vi "DriverStationGetData.vi"   [LabVIEW 2020]
doc: "This VI recieves data from the FRC 4265 Dashboard continuously, in all robot modes. These may include safety overrides, calibration commands, and configuration parameters. However this VI should never include standard driver or manipulator commands."
uses:
  f2972b46-d919-4210-bfdf-d3cf9c7f3ddc.vi
  <vilib>/Rock Robotics/Network Tables/NT Read Boolean.vi
  driverdata.vi
  <vilib>/Rock Robotics/Network Tables/NT Read Number.vi
  sensordata.vi
  <vilib>/Rock Robotics/Network Tables/NT Read Numeric Array.vi
  refnumbers.vi
  GRNF_Joystick.vi
  <vilib>/Rock Robotics/Network Tables/NT Read String.vi
  <vilib>/Utility/xml.llb/Write to XML File(string).vi
types:
  T1 = enum16{"Center", "North", "NorthWest", "West", "SouthWest", "South", "SouthEast", "East", "NorthEast"}
  T2 = typedef "WPI_JoystickDevRef.ctl" = cluster{"Device":T3}
  T3 = typedef "WPI_JoystickDeviceEnum.ctl" = enum16{"USB 0", "USB 1", "USB 2", "USB 3", "USB 4", "USB 5"}
  T4 = typedef "WPI_DriverStationAllianceInfo.ctl" = enum16{"Red", "Blue", "Invalid"}
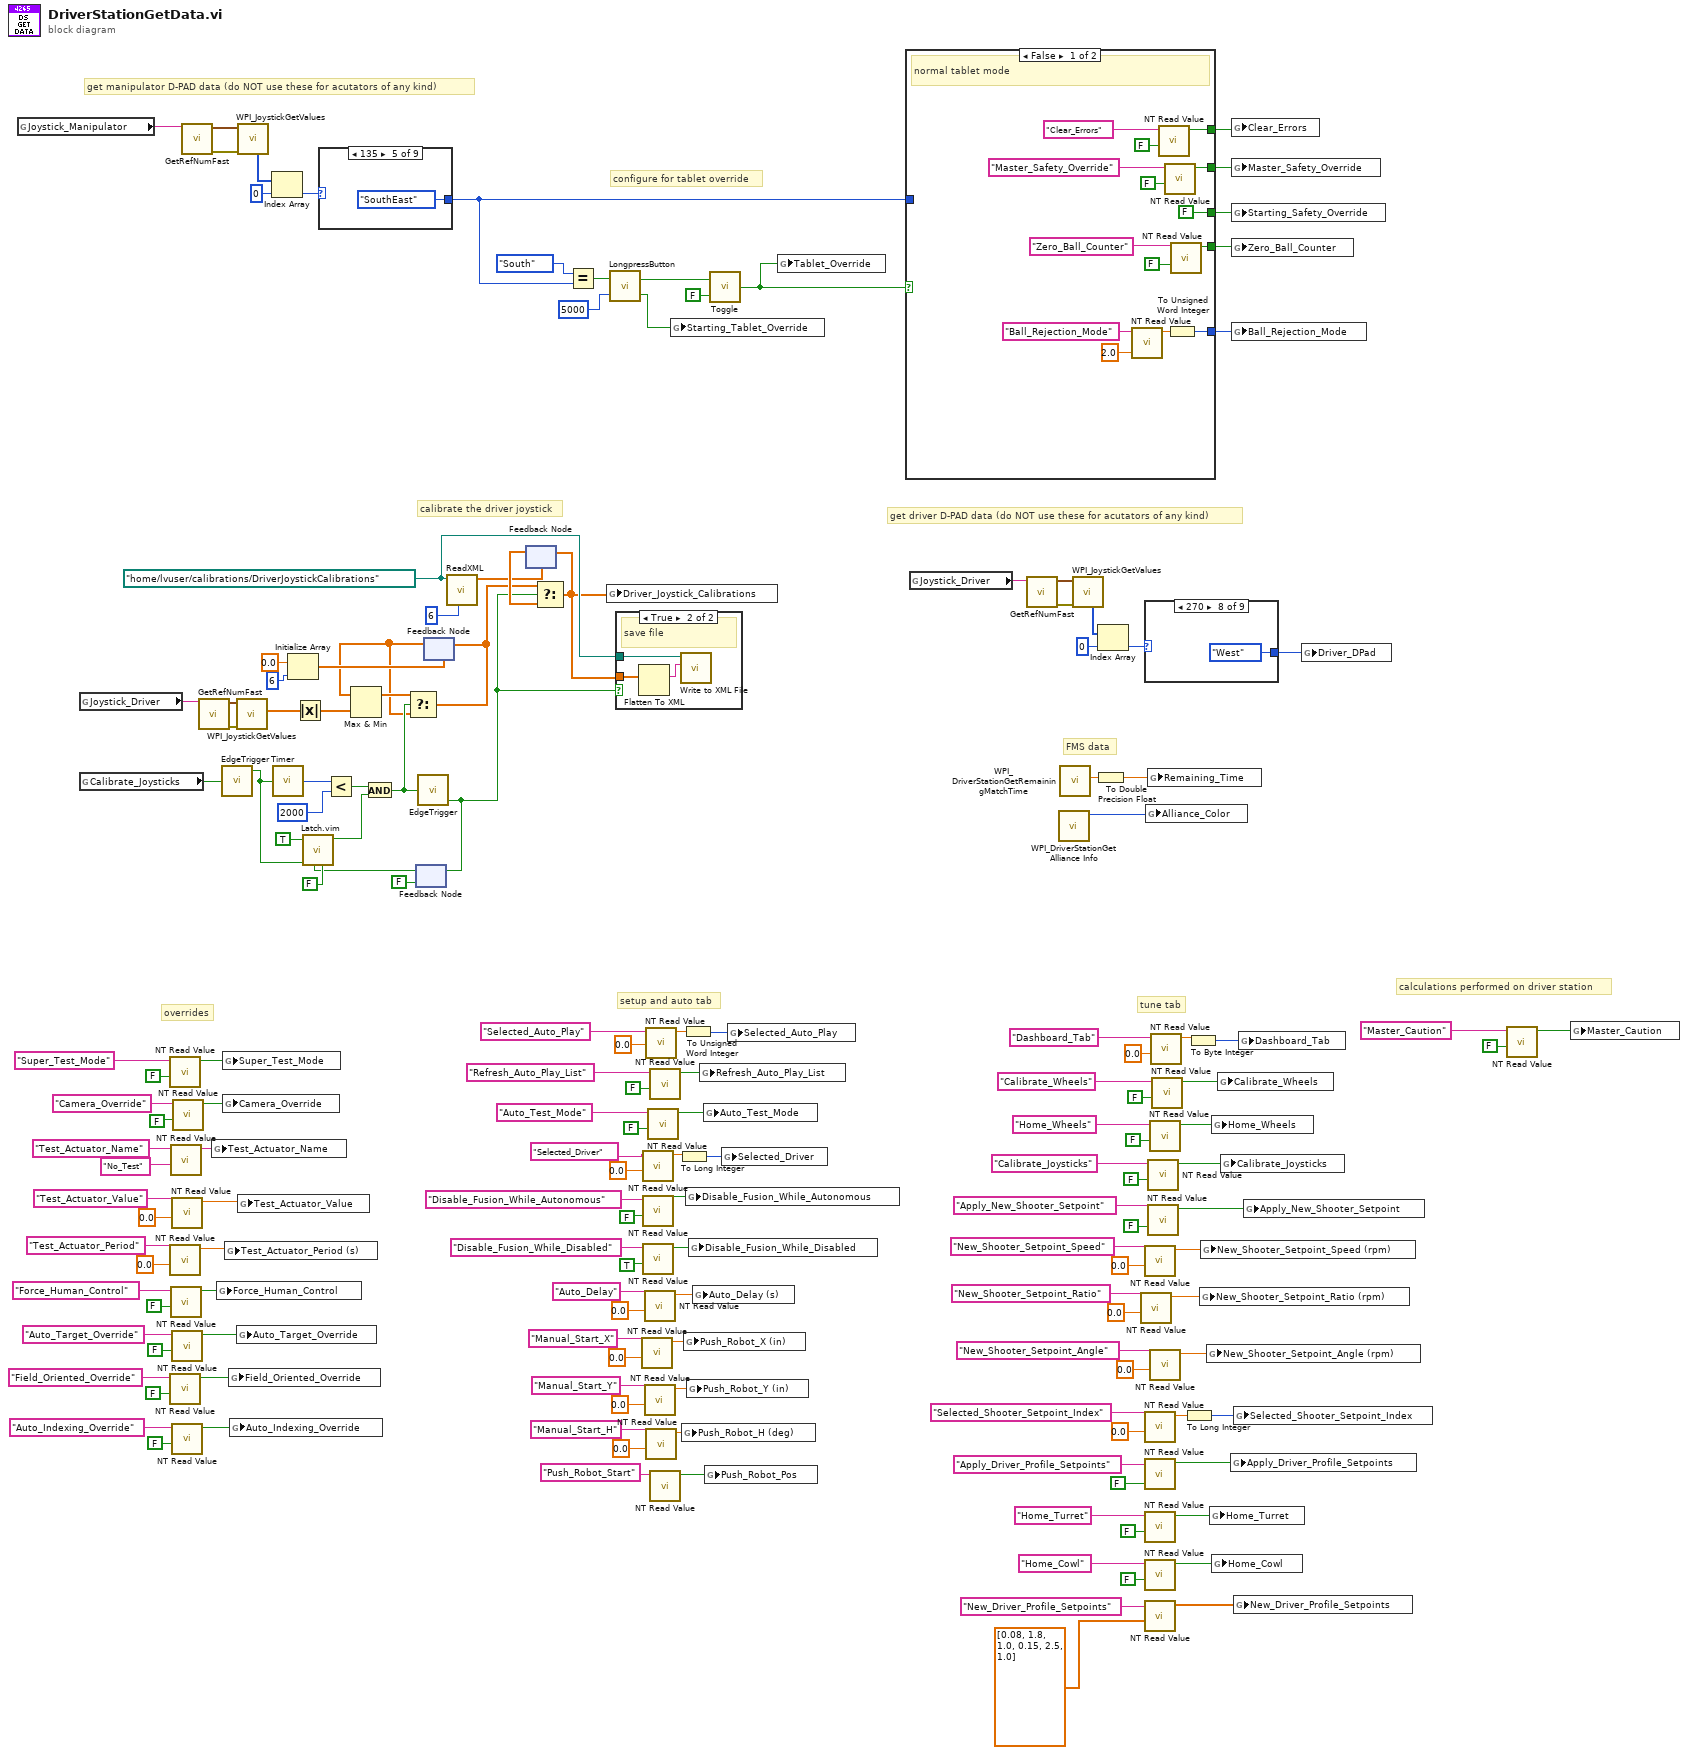
[diagram p0: block diagram]
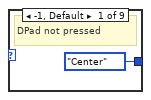
[diagram p2: hidden frame]
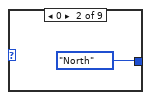
[diagram p3: hidden frame]
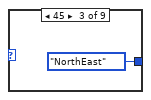
[diagram p4: hidden frame]
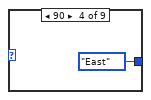
[diagram p5: hidden frame]
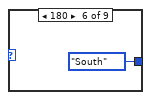
[diagram p6: hidden frame]
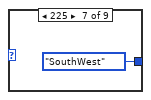
[diagram p7: hidden frame]
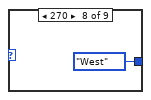
[diagram p8: hidden frame]
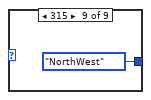
[diagram p9: hidden frame]
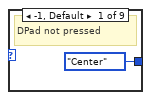
[diagram p10: hidden frame]
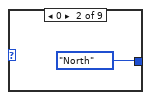
[diagram p11: hidden frame]
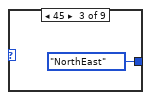
[diagram p12: hidden frame]
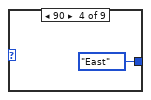
[diagram p13: hidden frame]
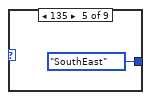
[diagram p14: hidden frame]
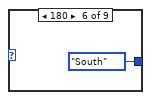
[diagram p15: hidden frame]
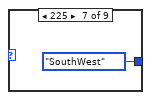
[diagram p16: hidden frame]
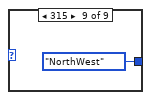
[diagram p17: hidden frame]
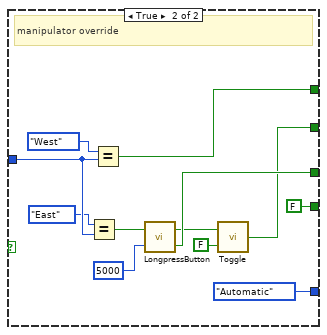
[diagram p19: hidden frame]
diagram:
  w100 = path "/home/lvuser/calibrations/DriverJoystickCalibrations" ("path")
  # "FMS data"
  # "get manipulator D-PAD data (do NOT use these for acutators of any kind)"
  # "get driver D-PAD data (do NOT use these for acutators of any kind)"
  # "calibrate the driver joystick"
  # "calculations performed on driver station"
  # "tune tab"
  # "overrides"
  # "setup and auto tab"
  # "configure for tablet override"
  n1 = global read "refnumbers.vi" "Joystick_Manipulator"() -> (w112:string)
  n2 = global read "refnumbers.vi" "Joystick_Driver"() -> (w96:string)
  n3 = global read "driverdata.vi" "Calibrate_Joysticks"() -> (w93:bool)
  n4 = call-poly <vilib>:"NT Read Value.vi"("Default Value"=FALSE, "Name"="Super_Test_Mode" ("refnum name")) -> ("Boolean"=w160:bool)  [unwired: 8 in, 1 out]
  n5 = call-poly <vilib>:"NT Read Value.vi"("Default Value"=0.0, "Name"="Test_Actuator_Period" ("refnum name")) -> ("Numeric"=w69:dbl)  [unwired: 8 in, 1 out]
  n6 = call-poly <vilib>:"NT Read Value.vi"("Default Value"=FALSE, "Name"="Field_Oriented_Override" ("refnum name")) -> ("Boolean"=w55:bool)  [unwired: 8 in, 1 out]
  n7 = call-poly <vilib>:"NT Read Value.vi"("Default Value"="No_Test", "Name"="Test_Actuator_Name" ("refnum name")) -> ("String"=w126:string)  [unwired: 8 in, 1 out]
  n8 = call-poly <vilib>:"NT Read Value.vi"("Default Value"=FALSE, "Name"="Force_Human_Control" ("refnum name")) -> ("Boolean"=w65:bool)  [unwired: 8 in, 1 out]
  n9 = call-poly <vilib>:"NT Read Value.vi"("Default Value"=0.0, "Name"="Test_Actuator_Value" ("refnum name")) -> ("Numeric"=w122:dbl)  [unwired: 8 in, 1 out]
  n10 = call-poly <vilib>:"NT Read Value.vi"("Default Value"=FALSE, "Name"="Auto_Target_Override" ("refnum name")) -> ("Boolean"=w119:bool)  [unwired: 8 in, 1 out]
  n11 = call-poly <vilib>:"NT Read Value.vi"("Default Value"=FALSE, "Name"="Auto_Indexing_Override" ("refnum name")) -> ("Boolean"=w2:bool)  [unwired: 8 in, 1 out]
  n12 = call-poly <vilib>:"NT Read Value.vi"("Default Value"=FALSE, "Name"="Camera_Override" ("refnum name")) -> ("Boolean"=w134:bool)  [unwired: 8 in, 1 out]
  n13 = call-poly "GetRefNumFast.vi"("RefNum Name"=w112) -> ("Error"=w113:errorcluster, "Device Reference"=w114:T2)  [unwired: 5 in]
  n14 = call-poly "GetRefNumFast.vi"("RefNum Name"=w96) -> ("Error"=w94:errorcluster, "Device Reference"=w95:T2)  [unwired: 5 in]
  n15 = global write "driverdata.vi" "Test_Actuator_Name"(w126) -> ()
  n16 = global write "driverdata.vi" "Force_Human_Control"(w65) -> ()
  n17 = call "EdgeTrigger.vi"("Input Signal"=w93) -> ("Rising Edge Trigger"=w92:bool)  [unwired: 2 out]
  n18 = global write "driverdata.vi" "Super_Test_Mode"(w160) -> ()
  n19 = global write "driverdata.vi" "Camera_Override"(w134) -> ()
  n20 = global write "driverdata.vi" "Test_Actuator_Period (s)"(w69) -> ()
  n21 = global write "driverdata.vi" "Field_Oriented_Override"(w55) -> ()
  n22 = global write "driverdata.vi" "Auto_Indexing_Override"(w2) -> ()
  n23 = call <vilib>:"WPI_JoystickGetValues.vi"("error in (no error)"=w94, "JoystickDevRef"=w95) -> ("Axes"=w80:dbl[])  [unwired: 5 in, 4 out]
  n24 = global write "driverdata.vi" "Auto_Target_Override"(w119) -> ()
  n25 = call <vilib>:"WPI_JoystickGetValues.vi"("error in (no error)"=w113, "JoystickDevRef"=w114) -> ("POVs"=w43:i16[])  [unwired: 5 in, 4 out]
  n26 = global write "driverdata.vi" "Test_Actuator_Value"(w122) -> ()
  n27 = Index Array(array=w43, index=0) -> (element=w44:i16)
  n28 = call "Timer.vi"("Reset Timer"=w92) -> ("Time (ms)"=w98:u32)
  n29 = Initialize Array(0.0 ("element"), 6 ("dimension size")) -> (w73:dbl[])
  n30 = Absolute Value(x=w80) -> (abs(x)=w77:dbl[])
  n31 = case shown="135" w44 {
    tunnel: [T1."Center" T1."North" T1."NorthEast" T1."East" T1."SouthEast" T1."South" T1."SouthWest" T1."West" T1."NorthWest"] -> w36
    frame -1, Default {
      # "DPad not pressed"
    }
    frame 0 {
    }
    frame 45 {
    }
    frame 90 {
    }
    frame 135 {
    }
    frame 180 {
    }
    frame 225 {
    }
    frame 270 {
    }
    frame 315 {
    }
  }
  n32 = Less?(x=w98, y=u32 2000) -> (x < y?=w89:bool)
  n33 = feedback #1(FALSE ("Falling Edge Trigger")) -> (w86:bool)
  n34 = call "Latch.vim"("Default Value"=FALSE, "Reset"=w86, "Latch Signal"=w92, "Latch Value"=TRUE) -> ("Latched"=w88:bool)  [unwired: 7 in]
  n35 = And(x=w89, y=w88) -> (x .and. y?=w87:bool)
  n36 = call "EdgeTrigger.vi"("Input Signal"=w87) -> ("Falling Edge Trigger"=w84:bool)  [unwired: 2 out]
  n37 = feedback-in #1(w84) -> ()
  n38 = feedback #2(w73) -> (w72:dbl[])
  n39 = Max & Min(x=w72, y=w77) -> (max(x,y)=w79:dbl[])  [unwired: 1 out]
  n40 = Select(t=w79, s=w87, f=w72) -> (s? t:f=w78:dbl[])
  n41 = feedback-in #2(w78) -> ()
  n42 = call "ReadXML.vi"("Default Number of Elements"=6, "File Path (.xml)"=w100) -> ("Data"=w99:dbl[])  [unwired: 8 in, 1 out]
  n43 = feedback #3(w99) -> (w101:dbl[])
  n44 = Select(t=w78, s=w84, f=w101) -> (s? t:f=w81:dbl[])
  n45 = feedback-in #3(w81) -> ()
  n46 = Equal?(x=T1."South", y=w36) -> (x = y?=w41:bool)
  n47 = global write "driverdata.vi" "Driver_Joystick_Calibrations"(w81) -> ()
  n48 = call "LongpressButton.vi"("Threshold (ms)"=u32 5000, "Button"=w41) -> ("Starting Press"=w35:bool, "Longpress Button"=w38:bool)
  n49 = case shown="True" w84 {
    tunnel: w100 -> [_ w174]
    tunnel: w81 -> [_ w173]
    frame False {
    }
    frame True {
      # "save file"
      n50 = Flatten To XML(6:w173) -> (2:w172:string)
      n51 = call-poly <vilib>:"Write to XML File.vi"("XML Input"=w172, "XML File Path"=w174) -> ()  [unwired: 7 in, 3 out]
    }
  }
  n52 = call-poly <vilib>:"NT Read Value.vi"("Default Value"=0.0, "Name"="Manual_Start_X" ("refnum name")) -> ("Numeric"=w109:dbl)  [unwired: 8 in, 1 out]
  n53 = call-poly <vilib>:"NT Read Value.vi"("Default Value"=0.0, "Name"="Selected_Driver" ("refnum name")) -> ("Numeric"=w150:dbl)  [unwired: 8 in, 1 out]
  n54 = call-poly <vilib>:"NT Read Value.vi"("Default Value"=FALSE, "Name"="Disable_Fusion_While_Autonomous" ("refnum name")) -> ("Boolean"=w131:bool)  [unwired: 8 in, 1 out]
  n55 = call-poly <vilib>:"NT Read Value.vi"("Default Value"=TRUE, "Name"="Disable_Fusion_While_Disabled" ("refnum name")) -> ("Boolean"=w128:bool)  [unwired: 8 in, 1 out]
  n56 = call-poly <vilib>:"NT Read Value.vi"("Default Value"=0.0, "Name"="Auto_Delay" ("refnum name")) -> ("Numeric"=w139:dbl)  [unwired: 8 in, 1 out]
  n57 = call-poly <vilib>:"NT Read Value.vi"("Default Value"=0.0, "Name"="Manual_Start_Y" ("refnum name")) -> ("Numeric"=w106:dbl)  [unwired: 8 in, 1 out]
  n58 = call-poly <vilib>:"NT Read Value.vi"("Default Value"=0.0, "Name"="Selected_Auto_Play" ("refnum name")) -> ("Numeric"=w154:dbl)  [unwired: 8 in, 1 out]
  n59 = call-poly <vilib>:"NT Read Value.vi"("Default Value"=0.0, "Name"="Manual_Start_H" ("refnum name")) -> ("Numeric"=w103:dbl)  [unwired: 8 in, 1 out]
  n60 = call-poly <vilib>:"NT Read Value.vi"("Default Value"=FALSE, "Name"="Auto_Test_Mode" ("refnum name")) -> ("Boolean"=w71:bool)  [unwired: 8 in, 1 out]
  n61 = call-poly <vilib>:"NT Read Value.vi"("Default Value"=FALSE, "Name"="Refresh_Auto_Play_List" ("refnum name")) -> ("Boolean"=w157:bool)  [unwired: 8 in, 1 out]
  n62 = call-poly <vilib>:"NT Read Value.vi"("Name"="Push_Robot_Start" ("refnum name")) -> ("Boolean"=w102:bool)  [unwired: 9 in, 1 out]
  n63 = global write "driverdata.vi" "Starting_Tablet_Override"(w35) -> ()
  n64 = To Long Integer(number=w150) -> (32bit integer=w148:i32)
  n65 = global write "sensordata.vi" "Push_Robot_H (deg)"(w103) -> ()
  n66 = To Unsigned Word Integer(number=w154) -> (unsigned 16bit integer=w153:u16)
  n67 = global write "sensordata.vi" "Push_Robot_X (in)"(w109) -> ()
  n68 = global write "driverdata.vi" "Disable_Fusion_While_Autonomous"(w131) -> ()
  n69 = global write "sensordata.vi" "Push_Robot_Y (in)"(w106) -> ()
  n70 = global write "driverdata.vi" "Disable_Fusion_While_Disabled"(w128) -> ()
  n71 = global write "driverdata.vi" "Auto_Delay (s)"(w139) -> ()
  n72 = global write "driverdata.vi" "Refresh_Auto_Play_List"(w157) -> ()
  n73 = global write "driverdata.vi" "Auto_Test_Mode"(w71) -> ()
  n74 = global write "sensordata.vi" "Push_Robot_Pos"(w102) -> ()
  n75 = call "Toggle.vi"("Initial State"=FALSE, "Trigger"=w38) -> ("New State"=w37:bool)
  n76 = global write "driverdata.vi" "Selected_Driver"(w148) -> ()
  n77 = global write "driverdata.vi" "Selected_Auto_Play"(w153) -> ()
  n78 = global write "driverdata.vi" "Tablet_Override"(w37) -> ()
  n79 = case shown="False" w37 {
    tunnel: [w186 w199] -> w118
    tunnel: w36 -> [_ w198]
    tunnel: [w183 w191] -> w34
    tunnel: [FALSE ("Starting Press") w194] -> w33
    tunnel: [w179 FALSE ("Boolean")] -> w5
    tunnel: [w175 enum16{"Theirs", "Automatic", "Ours"}."Automatic" ("Ball_Rejection_Mode")] -> w1
    frame False {
      # "normal tablet mode"
      n80 = call-poly <vilib>:"NT Read Value.vi"("Default Value"=2.0, "Name"="Ball_Rejection_Mode" ("refnum name")) -> ("Numeric"=w176:dbl)  [unwired: 8 in, 1 out]
      n81 = call-poly <vilib>:"NT Read Value.vi"("Default Value"=FALSE, "Name"="Clear_Errors" ("refnum name")) -> ("Boolean"=w186:bool)  [unwired: 8 in, 1 out]
      n82 = call-poly <vilib>:"NT Read Value.vi"("Default Value"=FALSE, "Name"="Master_Safety_Override" ("refnum name")) -> ("Boolean"=w183:bool)  [unwired: 8 in, 1 out]
      n83 = To Unsigned Word Integer(number=w176) -> (unsigned 16bit integer=w175:u16)
      n84 = call-poly <vilib>:"NT Read Value.vi"("Default Value"=FALSE, "Name"="Zero_Ball_Counter" ("refnum name")) -> ("Boolean"=w179:bool)  [unwired: 8 in, 1 out]
    }
    frame True {
      # "manipulator override"
      n85 = Equal?(x=T1."East", y=w198) -> (x = y?=w196:bool)
      n86 = Equal?(x=T1."West", y=w198) -> (x = y?=w199:bool)
      n87 = call "LongpressButton.vi"("Threshold (ms)"=u32 5000, "Button"=w196) -> ("Starting Press"=w194:bool, "Longpress Button"=w193:bool)
      n88 = call "Toggle.vi"("Initial State"=FALSE, "Trigger"=w193) -> ("New State"=w191:bool)
    }
  }
  n89 = global read "refnumbers.vi" "Joystick_Driver"() -> (w62:string)
  n90 = call-poly "GetRefNumFast.vi"("RefNum Name"=w62) -> ("Error"=w63:errorcluster, "Device Reference"=w64:T2)  [unwired: 5 in]
  n91 = call <vilib>:"WPI_DriverStationGet Alliance Info.vi"() -> ("Alliance"=w8:T4)  [unwired: 6 in, 5 out]
  n92 = call <vilib>:"WPI_DriverStationGetRemainingMatchTime.vi"() -> ("Match Time(s)"=w10:sgl)  [unwired: 10 in, 1 out]
  n93 = call <vilib>:"WPI_JoystickGetValues.vi"("error in (no error)"=w63, "JoystickDevRef"=w64) -> ("POVs"=w59:i16[])  [unwired: 5 in, 4 out]
  n94 = To Double Precision Float(number=w10) -> (double precision float=w9:dbl)
  n95 = Index Array(array=w59, index=0) -> (element=w60:i16)
  n96 = call-poly <vilib>:"NT Read Value.vi"("Default Value"=0.0, "Name"="New_Shooter_Setpoint_Ratio" ("refnum name")) -> ("Numeric"=w17:dbl)  [unwired: 8 in, 1 out]
  n97 = case shown="270" w60 {
    tunnel: [T1."Center" T1."North" T1."NorthEast" T1."East" T1."SouthEast" T1."South" T1."SouthWest" T1."West" T1."NorthWest"] -> w58
    frame -1, Default {
      # "DPad not pressed"
    }
    frame 0 {
    }
    frame 45 {
    }
    frame 90 {
    }
    frame 135 {
    }
    frame 180 {
    }
    frame 225 {
    }
    frame 270 {
    }
    frame 315 {
    }
  }
  n98 = call-poly <vilib>:"NT Read Value.vi"("Default Value"=0.0, "Name"="New_Shooter_Setpoint_Speed" ("refnum name")) -> ("Numeric"=w51:dbl)  [unwired: 8 in, 1 out]
  n99 = call-poly <vilib>:"NT Read Value.vi"("Default Value"=0.0, "Name"="Selected_Shooter_Setpoint_Index" ("refnum name")) -> ("Numeric"=w48:dbl)  [unwired: 8 in, 1 out]
  n100 = call-poly <vilib>:"NT Read Value.vi"("Default Value"=FALSE, "Name"="Apply_Driver_Profile_Setpoints") -> ("Boolean"=w30:bool)  [unwired: 8 in, 1 out]
  n101 = call-poly <vilib>:"NT Read Value.vi"("Default Value"=FALSE, "Name"="Home_Turret" ("refnum name")) -> ("Boolean"=w23:bool)  [unwired: 8 in, 1 out]
  n102 = call-poly <vilib>:"NT Read Value.vi"("Default Value"=FALSE, "Name"="Home_Cowl" ("refnum name")) -> ("Boolean"=w20:bool)  [unwired: 8 in, 1 out]
  n103 = call-poly <vilib>:"NT Read Value.vi"("Default Value"=dbl[] [0.08, 1.8, 1.0, 0.15, 2.5, 1.0], "Name"="New_Driver_Profile_Setpoints") -> ("Numeric Array"=w28:dbl[])  [unwired: 8 in, 1 out]
  n104 = global write "driverdata.vi" "Alliance_Color"(w8) -> ()
  n105 = global write "driverdata.vi" "Remaining_Time"(w9) -> ()
  n106 = call-poly <vilib>:"NT Read Value.vi"("Default Value"=FALSE, "Name"="Calibrate_Joysticks" ("refnum name")) -> ("Boolean"=w6:bool)  [unwired: 8 in, 1 out]
  n107 = call-poly <vilib>:"NT Read Value.vi"("Default Value"=FALSE, "Name"="Apply_New_Shooter_Setpoint" ("refnum name")) -> ("Boolean"=w7:bool)  [unwired: 8 in, 1 out]
  n108 = call-poly <vilib>:"NT Read Value.vi"("Default Value"=FALSE, "Name"="Home_Wheels" ("refnum name")) -> ("Boolean"=w26:bool)  [unwired: 8 in, 1 out]
  n109 = call-poly <vilib>:"NT Read Value.vi"("Default Value"=0.0, "Name"="New_Shooter_Setpoint_Angle" ("refnum name")) -> ("Numeric"=w14:dbl)  [unwired: 8 in, 1 out]
  n110 = call-poly <vilib>:"NT Read Value.vi"("Default Value"=0.0, "Name"="Dashboard_Tab" ("refnum name")) -> ("Numeric"=w12:dbl)  [unwired: 8 in, 1 out]
  n111 = call-poly <vilib>:"NT Read Value.vi"("Default Value"=FALSE, "Name"="Calibrate_Wheels" ("refnum name")) -> ("Boolean"=w145:bool)  [unwired: 8 in, 1 out]
  n112 = To Long Integer(number=w48) -> (32bit integer=w46:i32)
  n113 = To Byte Integer(number=w12) -> (8bit integer=w11:i8)
  n114 = global write "driverdata.vi" "New_Shooter_Setpoint_Ratio (rpm)"(w17) -> ()
  n115 = global write "driverdata.vi" "New_Shooter_Setpoint_Speed (rpm)"(w51) -> ()
  n116 = global write "driverdata.vi" "New_Shooter_Setpoint_Angle (rpm)"(w14) -> ()
  n117 = global write "driverdata.vi" "Home_Turret"(w23) -> ()
  n118 = global write "driverdata.vi" "Home_Wheels"(w26) -> ()
  n119 = global write "driverdata.vi" "Home_Cowl"(w20) -> ()
  n120 = global write "driverdata.vi" "Calibrate_Wheels"(w145) -> ()
  n121 = global write "driverdata.vi" "Calibrate_Joysticks"(w6) -> ()
  n122 = global write "driverdata.vi" "Apply_Driver_Profile_Setpoints"(w30) -> ()
  n123 = global write "driverdata.vi" "Clear_Errors"(w118) -> ()
  n124 = global write "driverdata.vi" "Master_Safety_Override"(w34) -> ()
  n125 = global write "driverdata.vi" "Starting_Safety_Override"(w33) -> ()
  n126 = global write "driverdata.vi" "Zero_Ball_Counter"(w5) -> ()
  n127 = global write "driverdata.vi" "Ball_Rejection_Mode"(w1) -> ()
  n128 = global write "driverdata.vi" "Selected_Shooter_Setpoint_Index"(w46) -> ()
  n129 = global write "driverdata.vi" "New_Driver_Profile_Setpoints"(w28) -> ()
  n130 = global write "driverdata.vi" "Dashboard_Tab"(w11) -> ()
  n131 = global write "driverdata.vi" "Apply_New_Shooter_Setpoint"(w7) -> ()
  n132 = global write "driverdata.vi" "Driver_DPad"(w58) -> ()
  n133 = call-poly <vilib>:"NT Read Value.vi"("Default Value"=FALSE, "Name"="Master_Caution" ("refnum name")) -> ("Boolean"=w115:bool)  [unwired: 8 in, 1 out]
  n134 = global write "driverdata.vi" "Master_Caution"(w115) -> ()
